vi "FPGA.vi"() -> ()   [LabVIEW 2013]
uses:
  <vilib>/rvi/FXPMathLib/FxpSinAndCos/XNode/nifxpmath_SinAndCos.xnode
  <vilib>/eio/EIONode/EIONode.xnode
  <vilib>/rvi/eio/common/nirviEmuTemplateMethod_errors.vi
  ToFPGA.ctl
  <vilib>/rvi/FXPMathLib/FxpSinAndCos/simVIs/DllFxpSinAndCosTemp_sub.vi
  <vilib>/rvi/FXPMathLib/FxpSinAndCos/subVIs/nifxpmath_SinAndCos_SimConfig.ctl
  FreqEstimator.ctl
  PMUmeasurements.ctl
panel:
  in  "Hold Time":sgl
  out "Loop period monitoring":u8
  in  "FPGA Loop \nTimer":u8 caption="Count(uSec)"
  out "output cluster":T1
  out "FPGA Error Out":errorcluster
  in  "alpha_Load":sgl
  in  "Scaling":sgl=80.0
  in  "Frequency Estimator Settings":T2={"Parameters"={"Ts"=5e-05, "kappaav"=0.625, "kappaph"=0.5762, "mu"=0.7086}}
  in  "Freq of Osc Load":sgl=0.64
  in  "PMU measurments":T3
  in  "stop":bool
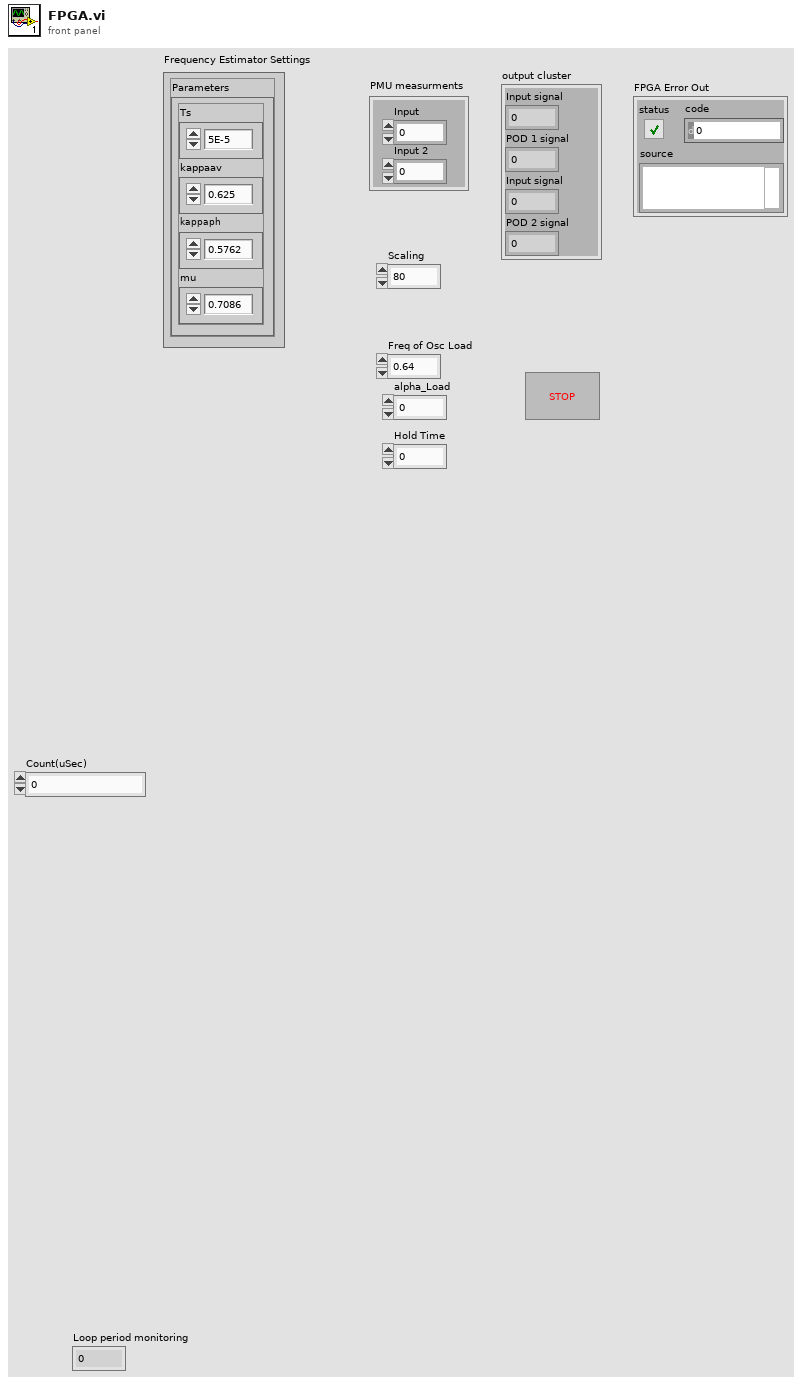
[diagram p1: front panel]
types:
  T1 = typedef "ToFPGA.ctl" = cluster{"Input signal":sgl, "POD 1 signal":sgl, "Input signal":sgl, "POD 2 signal":sgl}
  T2 = typedef "FreqEstimator.ctl" = cluster{"Parameters":cluster{"Ts":sgl, "kappaav":sgl, "kappaph":sgl, "mu":sgl}}
  T3 = typedef "PMUmeasurements.ctl" = cluster{"Input":sgl, "Input 2":sgl}
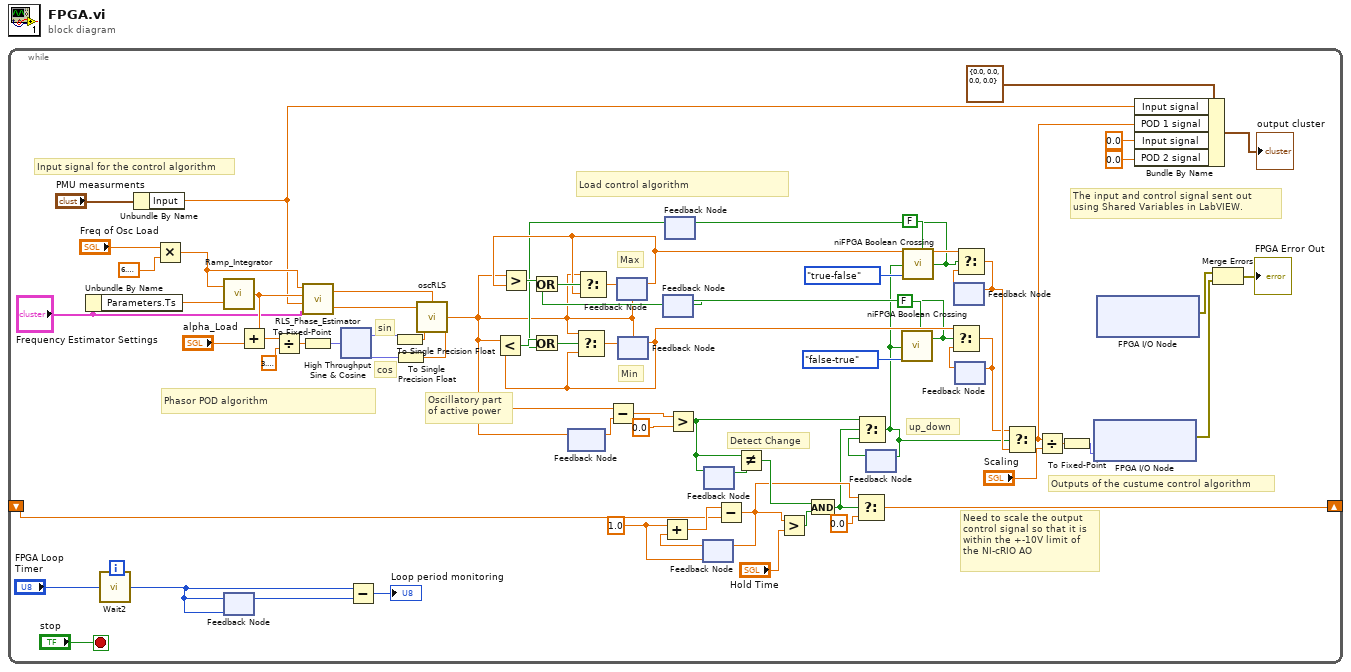
[diagram p0: block diagram]
diagram:
  n1 = while {
    shift-right: [w30] -> _
    shift-left: _ -> [w29]
    stop <- "stop" stop-if-true
    w36 = sgl 1.0 ("y")
    # "Need to scale the output \ncontrol signal so that it is \nwithin the +-10V limit of \nthe NI-cRIO AO"
    # "Load control algorithm"
    # "Phasor POD algorithm"
    # "Input signal for the control algorithm"
    # "The input and control signal sent out using Shared Variables in LabVIEW."
    # "Outputs of the custume control algorithm"
    # "up_down"
    # "Detect Change"
    # "Min"
    # "Max"
    # "Oscillatory part \nof active power"
    # "cos"
    # "sin"
    n2 = Unbundle By Name("Frequency Estimator Settings") -> ("Parameters.Ts"=w8:sgl)
    n3 = call "Wait2"("Count(uSec)"="FPGA Loop \nTimer") -> ("Tick Count(uSec)"=w40:u8)
    n4 = Unbundle By Name("PMU measurments") -> ("Input"=w6:sgl)
    n5 = Multiply(x="Freq of Osc Load", y=sgl 6.2831855) -> (x*y=w69:sgl)
    n6 = call "Ramp_Integrator.vi"("tsample"=w8, "w"=w69) -> ("theta"=w49:sgl)
    n7 = feedback #1(w40) -> (w42:u8)
    n8 = feedback-in #1(w40) -> ()
    n9 = Add(x=w49, y="alpha_Load") -> (x+y=w48:sgl)
    n10 = Divide(x=w48, y=sgl 3.1415927) -> (x/y=w67:sgl)
    n11 = call "RLS_Phase_Estimator.vi"("Frequency Estimator Settings"="Frequency Estimator Settings", "u"=w6, "theta"=w49, "wcs"=w69) -> ("uphq"=w60:sgl, "uphd"=w61:sgl)
    n12 = To Fixed-Point(number=w67) -> (fixed-point=w66:fxp<+/-,20,5>)  [unwired: 1 in]
    n13 = xnode "High Throughput Sine & Cosine"("x (pi)"=w66) -> ("sin(x)"=w65:fxp<+/-,16,2>, "cos(x)"=w64:fxp<+/-,16,2>)
    n14 = Subtract(x=w40, y=w42) -> (x-y=→"Loop period monitoring":u8)
    n15 = To Single Precision Float(number=w65) -> (single precision float=w63:sgl)
    n16 = To Single Precision Float(number=w64) -> (single precision float=w62:sgl)
    n17 = call "oscRLS.vi"("u4"=w63, "u3"=w62, "u2"=w60, "u1"=w61) -> ("f(u)"=w5:sgl)
    n18 = feedback #2() -> (w55:sgl)  [unwired: 1 in]
    n19 = feedback-in #2(w5) -> ()
    n20 = Subtract(x=w5, y=w55) -> (x-y=w53:sgl)
    n21 = feedback #3(w5) -> (w24:sgl)
    n22 = Greater?(x=w5, y=w24) -> (0:w59:bool)
    n23 = feedback #4(w5) -> (w23:sgl)
    n24 = Less?(x=w5, y=w23) -> (x < y?=w57:bool)
    n25 = feedback #5() -> (w15:bool)  [unwired: 1 in]
    n26 = Or(x=w59, y=w15) -> (x .or. y?=w58:bool)
    n27 = Select(t=w5, s=w58, f=w24) -> (s? t:f=w38:sgl)
    n28 = feedback-in #3(w38) -> ()
    n29 = feedback #6() -> (w17:bool)  [unwired: 1 in]
    n30 = Or(x=w57, y=w17) -> (x .or. y?=w56:bool)
    n31 = Select(t=w5, s=w56, f=w23) -> (s? t:f=w39:sgl)
    n32 = feedback-in #4(w39) -> ()
    n33 = Greater?(x=w53, y=sgl 0.0) -> (0:w28:bool)
    n34 = feedback #7(w36) -> (w37:sgl)
    n35 = Add(x=w36, y=w37) -> (x+y=w31:sgl)
    n36 = feedback #8(w28) -> (w33:bool)
    n37 = feedback-in #8(w28) -> ()
    n38 = Subtract(x=w31, y=w29) -> (x-y=w12:sgl)
    n39 = feedback-in #7(w12) -> ()
    n40 = Not Equal?(x=w28, y=w33) -> (x != y?=w13:bool)
    n41 = Greater?(x=w12, y="Hold Time") -> (0:w35:bool)
    n42 = And(x=w13, y=w35) -> (x .and. y?=w10:bool)
    n43 = Select(t=w12, s=w10, f=sgl 0.0) -> (s? t:f=w30:sgl)
    n44 = feedback #9() -> (w27:bool)  [unwired: 1 in]
    n45 = Select(t=w28, s=w10, f=w27) -> (s? t:f=w11:bool)
    n46 = feedback-in #9(w11) -> ()
    n47 = call <vilib>:"niFPGA Boolean Crossing.vi"("input"=w11, "direction"=enum8{"either", "false-true", "true-false"}."false-true", "initialize"=FALSE) -> ("crossing"=w16:bool)  [unwired: 6 in]
    n48 = feedback-in #5(w16) -> ()
    n49 = call <vilib>:"niFPGA Boolean Crossing.vi"("input"=w11, "direction"=enum8{"either", "false-true", "true-false"}."true-false", "initialize"=FALSE) -> ("crossing"=w18:bool)  [unwired: 6 in]
    n50 = feedback-in #6(w18) -> ()
    n51 = feedback #10() -> (w26:sgl)  [unwired: 1 in]
    n52 = feedback #11() -> (w25:sgl)  [unwired: 1 in]
    n53 = Select(t=w23, s=w16, f=w25) -> (s? t:f=w9:sgl)
    n54 = feedback-in #11(w9) -> ()
    n55 = Select(t=w24, s=w18, f=w26) -> (s? t:f=w14:sgl)
    n56 = feedback-in #10(w14) -> ()
    n57 = Select(t=w9, s=w11, f=w14) -> (s? t:f=w1:sgl)
    n58 = Divide(x=w1, y="Scaling") -> (x/y=w4:sgl)
    n59 = To Fixed-Point(number=w4) -> (fixed-point=w52:fxp<+/-,20,5>)  [unwired: 1 in]
    n60 = xnode "FPGA I/O Node"("Mod1/AO0"=w52) -> ("error out"=w46:errorcluster)  [unwired: 2 in, 1 out]
    n61 = xnode "FPGA I/O Node"() -> ("error out"=w47:errorcluster)  [unwired: 3 in, 1 out]
    n62 = Bundle By Name(cluster=T1 {"Input signal"=0.0, "POD 1 signal"=0.0, "Input signal"=0.0, "POD 2 signal"=0.0}, "Input signal"=w6, "POD 1 signal"=w1, "Input signal"=sgl 0.0 ("Empty"), "POD 2 signal"=sgl 0.0 ("Empty")) -> (→"output cluster":T1)
    n63 = Merge Errors(w47, w46) -> (→"FPGA Error Out":errorcluster)
  }
